vi "Notify Islanded.vi"(8 "error in (no error)":errorcluster, 11 "Master Controller in":refnum<class "Master Controller.lvclass">) -> (0 "error out":errorcluster, 3 "Master Controller out":refnum<class "Master Controller.lvclass">)   [LabVIEW 2015, in "Master Controller Core.lvlib" / "Master Controller.lvclass"]
uses:
  Master Controller.lvclass
  Communications/SCADA Communcations Actor/SCADA Communications/Controls/EMS Message Cluster.ctl
  Master Controller.lvclass/Master Controller.ctl
  Communications/SCADA Communcations Actor/SCADA Communications Messages/Transmit EMS Message Msg/Transmit EMS Message Msg.lvclass/Transmit EMS Message Msg.ctl
  <vilib>/ActorFramework/Message Enqueuer/Message Enqueuer.lvclass/Message Enqueuer.ctl
  <vilib>/ActorFramework/Message Enqueuer/Enqueue.vi
  <vilib>/ActorFramework/Message Priority Queue/Priority Enqueue.vi
  Communications/SCADA Communcations Actor/SCADA Communications Messages/Transmit EMS Message Msg/Transmit EMS Message Msg.lvclass
  Communications/SCADA Communcations Actor/SCADA Communications/SCADA Communications.lvclass
  Utilities/Status Messaging.llb/Status Messaging.lvlib
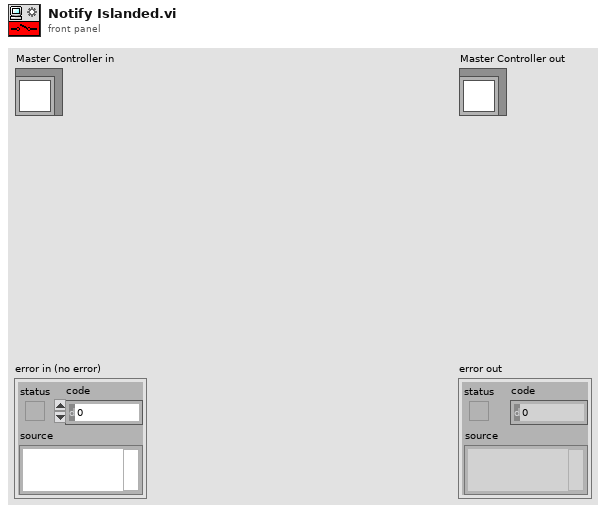
[diagram p1: front panel]
types:
  T1 = typedef "SCADA Communcations Actor.lvlib/SCADA Communications.lvclass/EMS Message Cluster.ctl" = cluster{"Name":string, "Content":string}
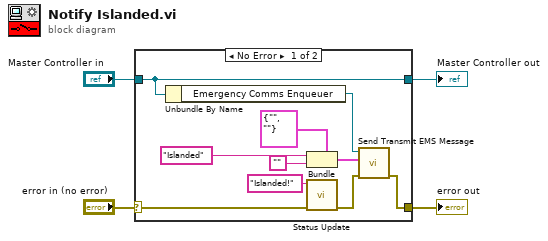
[diagram p0: block diagram]
diagram:
  n1 = case shown="No Error" "error in (no error)" {
    selector: "error in (no error)" -> [w7 w16]
    tunnel: [w9 w16] -> w2
    tunnel: [w10 w15] -> w3
    tunnel: "Master Controller in" -> [w10 w15]
    frame No Error {
      n2 = Unbundle By Name(w10) -> ("Emergency Comms Enqueuer"=w12:refnum<class "Message Enqueuer.lvclass">)
      n3 = Bundle(cluster=T1 {"Name"="", "Content"=""} ("Message"), "Name"="Islanded", "Content"="") -> (w13:T1)
      n4 = call "Status Update.vi"("error in (no error)"=w7, "Status Update"="Islanded!") -> ("error out"=w6:errorcluster)  [unwired: 8 in, 1 out]
      n5 = call "Send Transmit EMS Message.vi"("error in (no error)"=w6, "Message"=w13, "Message Enqueuer"=w12) -> ("error out"=w9:errorcluster)  [unwired: 7 in, 1 out]
    }
    frame Error {
    }
  }
  "error out" <- w2
  "Master Controller out" <- w3
